vi "gen field values.vi"(4 "x axis":string, 6 "Numeric 3":i32, 7 "Numeric":dbl, 9 "Auto x axis T":bool, 10 "Numeric 2":dbl, 11 "file path (dialog if empty)":path) -> (3 "1d Data":dbl[](array[numeric]))   [LabVIEW 2021]
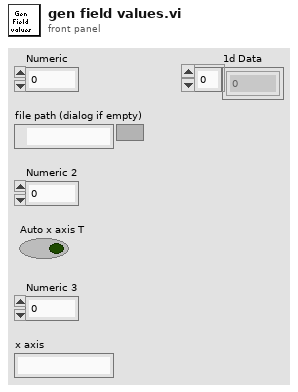
[diagram p1: front panel]
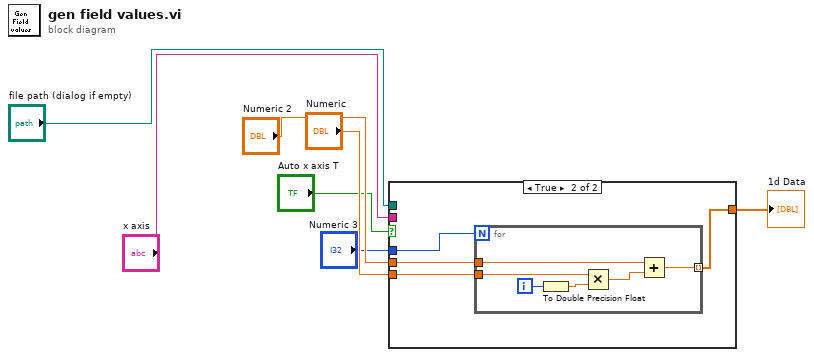
[diagram p0: block diagram]
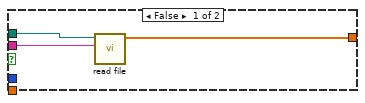
[diagram p2: hidden frame]
diagram:
  n1 = case shown="True" "Auto x axis T" {
    tunnel: [w8 w11] -> w2
    tunnel: "file path (dialog if empty)" -> [w10 _]
    tunnel: "x axis" -> [w9 _]
    tunnel: "Numeric 3" -> [_ w14]
    tunnel: "Numeric 2" -> [_ w13]
    tunnel: "Numeric" -> [_ w12]
    frame False {
      n2 = call "read file.vi"("file name"=w9, "file path (dialog if empty)"=w10) -> ("1d Data"=w8:dbl[])  [unwired: 8 in, 1 out]
    }
    frame True {
      n3 = for {
        N: w14 -> [_]
        tunnel: w13 -> [w20]
        tunnel: w12 -> [w18]
        tunnel: [w16] -> w11 mode=indexing
        i -> [w19]
        n4 = To Double Precision Float(number=w19) -> (double precision float=w15:dbl)
        n5 = Multiply(x=w18, y=w15) -> (x*y=w17:dbl)
        n6 = Add(x=w20, y=w17) -> (x+y=w16:dbl)
      }
    }
  }
  "1d Data" <- w2
